vi "remove_empty_files.vi"(8 "error in (no error)":errorcluster, 11 "ErrorController in":refnum<class "ErrorController.lvclass">) -> (0 "error out":errorcluster, 3 "ErrorController out":refnum<class "ErrorController.lvclass">)   [LabVIEW 2010, in "ErrorController.lvclass"]
uses:
  ErrorController.lvclass
  ErrorController.lvclass/ErrorController.ctl
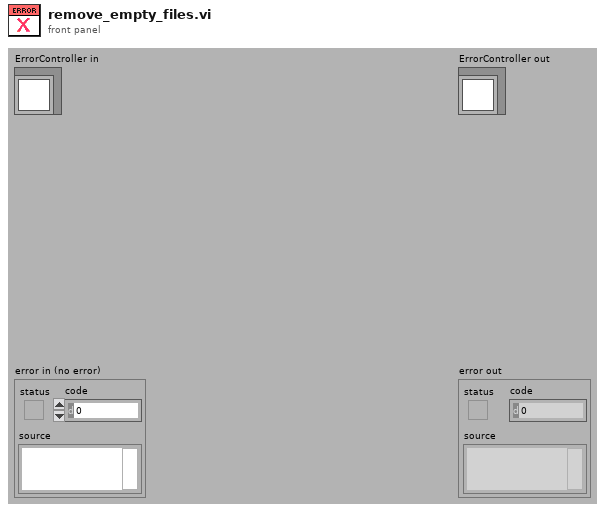
[diagram p1: front panel]
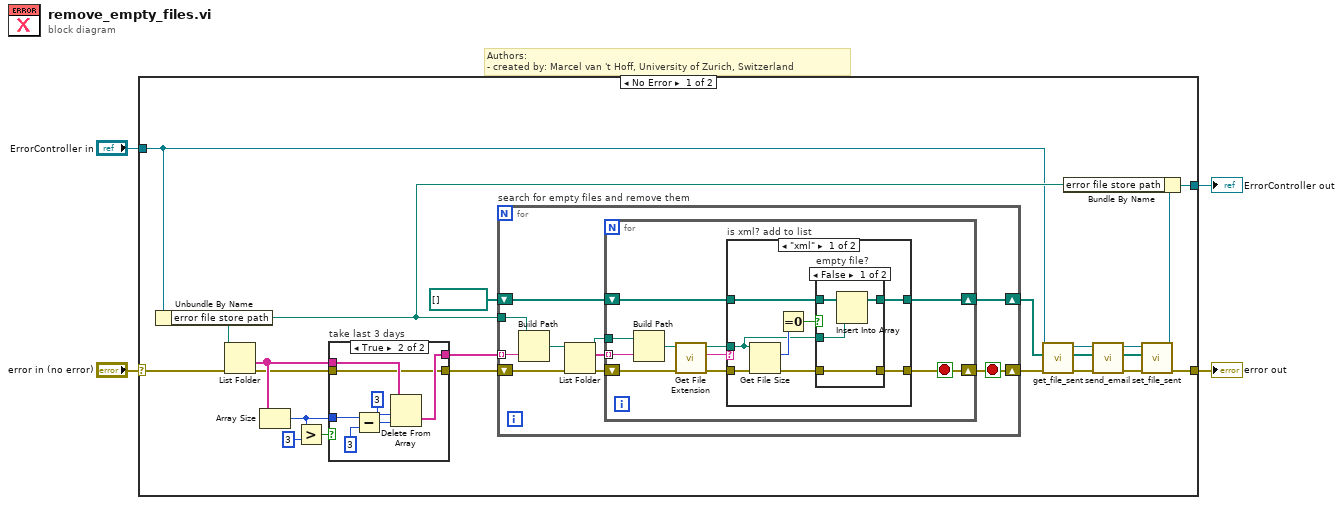
[diagram p0: block diagram]
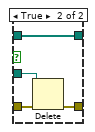
[diagram p3: hidden frame]
diagram:
  # "Authors: \n- created by: Marcel van 't Hoff, University of Zurich, Switzerland"
  n1 = case shown="No Error" "error in (no error)" {
    selector: "error in (no error)" -> [w26 w75]
    tunnel: [w24 w75] -> w3
    tunnel: [w7 w74] -> w1
    tunnel: "ErrorController in" -> [w6 w74]
    frame No Error {
      n2 = Unbundle By Name(w6) -> ("error file store path"=w8:path)
      n3 = List Folder(path=w8, error in=w26) -> (folder names=w15:string[], error out=w10:errorcluster)  [unwired: 2 in, 2 out]
      n4 = Array Size(array=w15) -> (size(s)=w13:i32)
      n5 = Greater?(x=w13, y=3) -> (0:w11:bool)
      n6 = case "take last 3 days" shown="True" w11 {
        tunnel: w13 -> [_ w35]
        tunnel: w15 -> [w28 w31]
        tunnel: [w28 w30] -> w14
        tunnel: w10 -> [w27 w29]
        tunnel: [w27 w29] -> w9
        frame False {
        }
        frame True {
          n7 = Subtract(x=w35, y=3) -> (x-y=w33:i32)
          n8 = Delete From Array(array=w31, length=3, index=w33) -> (deleted portion=w30:string[])  [unwired: 1 out]
        }
      }
      n9 = for "search for empty files and remove them" {
        tunnel: w14 -> [w42] mode=indexing
        shift-right: [w38] -> w16
        shift-left: path[] [] -> [w37]
        tunnel: w8 -> [w36]
        shift-right: [w43] -> w25
        shift-left: w9 -> [w45]
        stop <- w43 stop-if-true
        n10 = Build Path(base path=w36, name or relative path=w42) -> (appended path=w41:path)
        n11 = List Folder(path=w41, error in=w45) -> (path out=w39:path, filenames=w40:string[], error out=w44:errorcluster)  [unwired: 2 in, 1 out]
        n12 = for {
          tunnel: w40 -> [w54] mode=indexing
          tunnel: w39 -> [w53]
          shift-right: [w51] -> w38
          shift-left: w37 -> [w52]
          shift-right: [w55] -> w43
          shift-left: w44 -> [w50]
          stop <- w55 stop-if-true
          n13 = Build Path(base path=w53, name or relative path=w54) -> (appended path=w48:path)
          n14 = call <vilib>:"Get File Extension.vi"("error in (no error)"=w50, "file"=w48) -> ("error out"=w49:errorcluster, "lowercase file extension"=w46:string, "dup file"=w47:path)  [unwired: 6 in, 1 out]
          n15 = case "is xml? add to list" shown="\"xml\"" w46 {
            tunnel: [w63 w72] -> w55
            tunnel: w52 -> [w62 w73]
            tunnel: [w61 w73] -> w51
            tunnel: w49 -> [w57 w72]
            tunnel: w47 -> [w56 _]
            frame "xml" {
              n16 = Get File Size(file=w56, error in=w57) -> (size (in bytes)=w60:i64, 0:w58:errorcluster)  [unwired: 1 out]
              n17 = Equal To 0?(x=w60) -> (x = 0?=w59:bool)
              n18 = case "empty file?" shown="False" w59 {
                tunnel: w58 -> [w67 w71]
                tunnel: [w67 w70] -> w63
                tunnel: w62 -> [w66 w69]
                tunnel: [w65 w69] -> w61
                tunnel: w56 -> [w64 w68]
                frame False {
                  n19 = Insert Into Array(array=w66, new element=w64) -> (w65:path[])  [unwired: 1 in]
                }
                frame True {
                  n20 = Delete(path (use dialog)=w68, error in=w71) -> (error out=w70:errorcluster)  [unwired: 3 in, 2 out]
                }
              }
            }
            frame Default {
            }
          }
        }
      }
      n21 = call-dynamic "get_file_sent.vi"("error in (no error)"=w25, "path array in"=w16, "ErrorController in"=w6) -> ("error out"=w22:errorcluster, "path array out"=w20:path[], "ErrorController out"=w17:refnum<class "ErrorController.lvclass">)  [unwired: 6 in]
      n22 = call-dynamic "send_email.vi"("error in (no error)"=w22, "attachments array in"=w20, "ErrorController in"=w17) -> ("error out"=w21:errorcluster, "attachments array out"=w19:path[], "ErrorController out"=w18:refnum<class "ErrorController.lvclass">)  [unwired: 6 in]
      n23 = call-dynamic "set_file_sent.vi"("error in (no error)"=w21, "path array in"=w19, "ErrorController in"=w18) -> ("error out"=w24:errorcluster, "ErrorController out"=w5:refnum<class "ErrorController.lvclass">)  [unwired: 7 in]
      n24 = Bundle By Name(cluster=w5, "error file store path"=w8) -> (w7:refnum<class "ErrorController.lvclass">)
    }
    frame Error {
    }
  }
  "error out" <- w3
  "ErrorController out" <- w1
